vi "Navigation_Main_position_testing april 22.vi"() -> ()   [LabVIEW 2015]
uses:
  <vilib>/myRIO/Instrument Drivers/Onboard IO/PWM/typedefs/PWM Reference.ctl
  <vilib>/myRIO/Common/Instrument Driver Framework/Utilities/typedefs/myRIO Generic Hardware Reference.ctl
  <vilib>/myRIO/Common/Instrument Driver Framework/Utilities/typedefs/Hardware Version Enum.ctl
  <vilib>/myRIO/Common/Instrument Driver Framework/Utilities/typedefs/myRIO v1.0 Reference.ctl
  <vilib>/myRIO/Common/Instrument Driver Framework/Utilities/typedefs/Generic FPGA Reference.ctl
  <vilib>/myRIO/Common/Instrument Driver Framework/myRIO v1.0/PWM/typedefs/PWM Channels Enum.ctl
  <vilib>/myRIO/Instrument Drivers/Onboard IO/PWM/typedefs/PWM Configuration.ctl
  <vilib>/userdefined/High Color/nirio_resource_hc.ctl
  <vilib>/myRIO/Common/Instrument Driver Framework/myRIO v1.0/PWM/vis/myRIO v1.1 Open PWM.vi
  <vilib>/myRIO/Common/Instrument Driver Framework/Utilities/vis/Validate Channels.vi
  <vilib>/myRIO/Common/Instrument Driver Framework/myRIO v1.0/PWM/vis/myRIO v1.0 Reserve PWM.vi
  <vilib>/myRIO/Common/Instrument Driver Framework/myRIO v1.0/PWM/vis/myRIO v1.0 Build MUX Configuration PWM.vi
  <vilib>/myRIO/Common/Instrument Driver Framework/myRIO v1.0/Resource Manager/vis/myRIO v1.0 Reserve Channel List.vi
  <vilib>/myRIO/Common/Instrument Driver Framework/myRIO v1.0/Resource Manager/vis/myRIO v1.0 Create Configuration List.vi
  <vilib>/myRIO/Common/Instrument Driver Framework/myRIO v1.0/Resource Manager/vis/myRIO v1.0 Reserve Channel.vi
  <vilib>/myRIO/Common/Instrument Driver Framework/myRIO v1.0/Resource Manager/vis/myRIO v1.0 Unreserve Channel.vi
  <vilib>/myRIO/Common/Instrument Driver Framework/myRIO v1.0/Resource Manager/vis/myRIO v1.0 Build Mutex Name.vi
  <vilib>/FPGAPlugInAG/myRIO-1900/niLvFpga_Open_myRIO-1900.vi
  <vilib>/rvi/interface/common/dynamic/niFpgaDynamicAddResources.vi
  <vilib>/myRIO/Common/Instrument Driver Framework/Utilities/vis/FPGA Ref Manager.vi
  <vilib>/Utility/error.llb/Error Cluster From Error Code.vi
  <vilib>/myRIO/Common/Instrument Driver Framework/Utilities/vis/Ref Counter.vi
  <vilib>/rvi/errors/niLvFpgaAdjustHostInterfaceError.vi
  <vilib>/Utility/VariantDataType/GetNumericInfo.vi
  <vilib>/myRIO/Common/Instrument Driver Framework/myRIO v1.0/myRIO v1.1 Open.vi
  <vilib>/myRIO/Common/Instrument Driver Framework/Utilities/vis/IO Manager.vi
  <vilib>/myRIO/Common/Instrument Driver Framework/Utilities/vis/Configuration Manager.vi
  <vilib>/myRIO/Common/Instrument Driver Framework/myRIO v1.0/Resource Manager/vis/myRIO v1.0 Configure IO.vi
  <vilib>/myRIO/Common/Instrument Driver Framework/myRIO v1.0/myRIO v1.0 Close.vi
  <vilib>/myRIO/Common/Instrument Driver Framework/myRIO v1.0/PWM/vis/myRIO v1.0 Write PWM.vi
  <vilib>/addons/control/pid/pid.llb/PID (DBL).vi
  <vilib>/rvi/interface/nirviOpenFPGA/nirviOpenFPGA.xnode
  Navi/E/FPGA Bitfiles/NavigationProjec_FPGATarget2_FPGAMainNavigati_PWPHW8gwDxI.lvbitx
  <vilib>/rvi/interface/nirviReadWriteControl/nirviReadWriteControl.xnode
  <vilib>/myRIO/Instrument Drivers/Onboard IO/PWM/vis/myRIO PWM Open.xnode
  <vilib>/myRIO/Instrument Drivers/Onboard IO/PWM/PWM.lvlib
  <vilib>/myRIO/Instrument Drivers/Utilities/Utilities.lvlib
  NiFpgaLv.dll
  <vilib>/rvi/interface/Simulation/niFpgaSimulationCallBeginRW.vi
  <vilib>/addons/control/pid/NI_PID_pid.lvlib
panel:
  in  "camera drop out while loop":bool
  in  "mining control while loop":bool
  in  "Boolean 2":bool=TRUE
  out "stop switch":dbl=1.0
  out "distance to goal":dbl
  out "loc_y":dbl
  out "loc_x":dbl
  out "loc_theta":dbl
  out "start y":dbl
  out "start angle":dbl=1.0
  out "start x":dbl=1.0
  in  "set start position":bool=TRUE
  out "goal reached":bool=TRUE
  out "x/y":dbl
  out "scale":dbl=1.0
  in  "x goal":dbl=10.0
  in  "L Desired Input Velocity (ft/s) 4":dbl(knob) scale=-4.0..4.0
  in  "R Min Linear Velocity (ft/s)  2":dbl=-2.0 format="%#_13g"
  in  "L Min Linear Velocity (ft/s) 9":dbl=-2.0 format="%#_13g"
  in  "R Max Linear Velocity (ft/s) 5":dbl=2.0 format="%#_13g"
  in  "L Max Linear Velocity (ft/s) 5":dbl=2.0 format="%#_13g"
  in  "R Desired Input Velocity (ft/s) 5":dbl(knob) scale=-4.0..4.0
  out "left":dbl
  out "right":dbl
  out "left wheels actual pwm":dbl
  in  "pid reset left":bool
  out "left pwm":dbl(graph)
  out "dt out (s) 3":dbl format="%.3f"
  in  "output range 3":cluster{"output high":dbl, "output low":dbl}={"output high"=0.13333, "output low"=-0.13333} {"output low" format="%.6f"; "output high" format="%.5f"}
  in  "PID gains 3":T1={"proportional gain (Kc)"=0.002, "integral time (Ti, min)"=7e-07, "derivative time (Td, min)"=0.0} {"derivative time (Td, min)" format="%.8f"; "integral time (Ti, min)" format="%.8f"; "proportional gain (Kc)" format="%.8f"}
  out "desired pwm 2":dbl
  out "feedback 2":dbl
  out ".not. x? 3":bool
  out "Elapsed Time (s) 2":dbl caption="Elapsed Time (s)"
  out "x traveled 2":dbl
  out "y traveled 2":dbl
  out "avg 124":dbl
  out "avg 457":dbl
  out "psi dot 2":dbl
  out "distance traveled 2":dbl
  out "y dot 2":dbl
  out "x dot 2":dbl
  out "x position 2":dbl
  out "y position 2":dbl
  out "reset x y 2":dbl
  out "Tick Count(mSec) 2":u32 caption="Tick Count(mSec)"
  in  "start y 2":dbl=3.0
  in  "start x 2":dbl=1.0
  out "right wheels actual pwm":dbl
  in  "pid reset right":bool
  out "right pwm":dbl(graph)
  out "dt out (s) 2":dbl format="%.3f"
  in  "output range 2":cluster{"output high":dbl, "output low":dbl}={"output high"=0.13333, "output low"=-0.13333} {"output low" format="%.6f"; "output high" format="%.5f"}
  in  "PID gains 2":T1={"proportional gain (Kc)"=0.002, "integral time (Ti, min)"=7e-07, "derivative time (Td, min)"=0.0} {"derivative time (Td, min)" format="%.8f"; "integral time (Ti, min)" format="%.8f"; "proportional gain (Kc)" format="%.8f"}
  out "desired pwm":dbl
  out "feedback":dbl
  out ".not. x? 2":bool
  out "Elapsed Time (s)":dbl
  out "LF Rot Velocity (rot/s)":dbl
  out "LM Rot Velocity (rot/s)":dbl
  out "LR Rot Velocity (rot/s)":dbl
  out "RR Rot Velocity (rot/s)":dbl
  out "RM Linear Velocity (rot/s)":dbl
  out "RF Linear Velocity (rot/s)":dbl
  in  "Encoder Reset":bool
  out "SYS.SELECTA":u8 format="%08b"
  out "ENC.B_c.CNTR":i32
  out "ENC.B_b.CNTR":i32
  out "ENC.B_a.CNTR":i32
  out "ENC.A_c.CNTR":i32
  out "ENC.A_b.CNTR":i32
  out "ENC.A_a.CNTR":i32
  in  "R Min Linear Velocity (ft/s)":dbl=-2.0 format="%#_13g"
  in  "R Max Linear Velocity (ft/s)":dbl=2.0 format="%#_13g"
  in  "L Min Linear Velocity (ft/s)":dbl=-2.0 format="%#_13g"
  in  "L Max Linear Velocity (ft/s)":dbl=2.0 format="%#_13g"
  out "Current Rot Velocity (rot/s)":T2(graph)
  # "Motor Control Parameters"
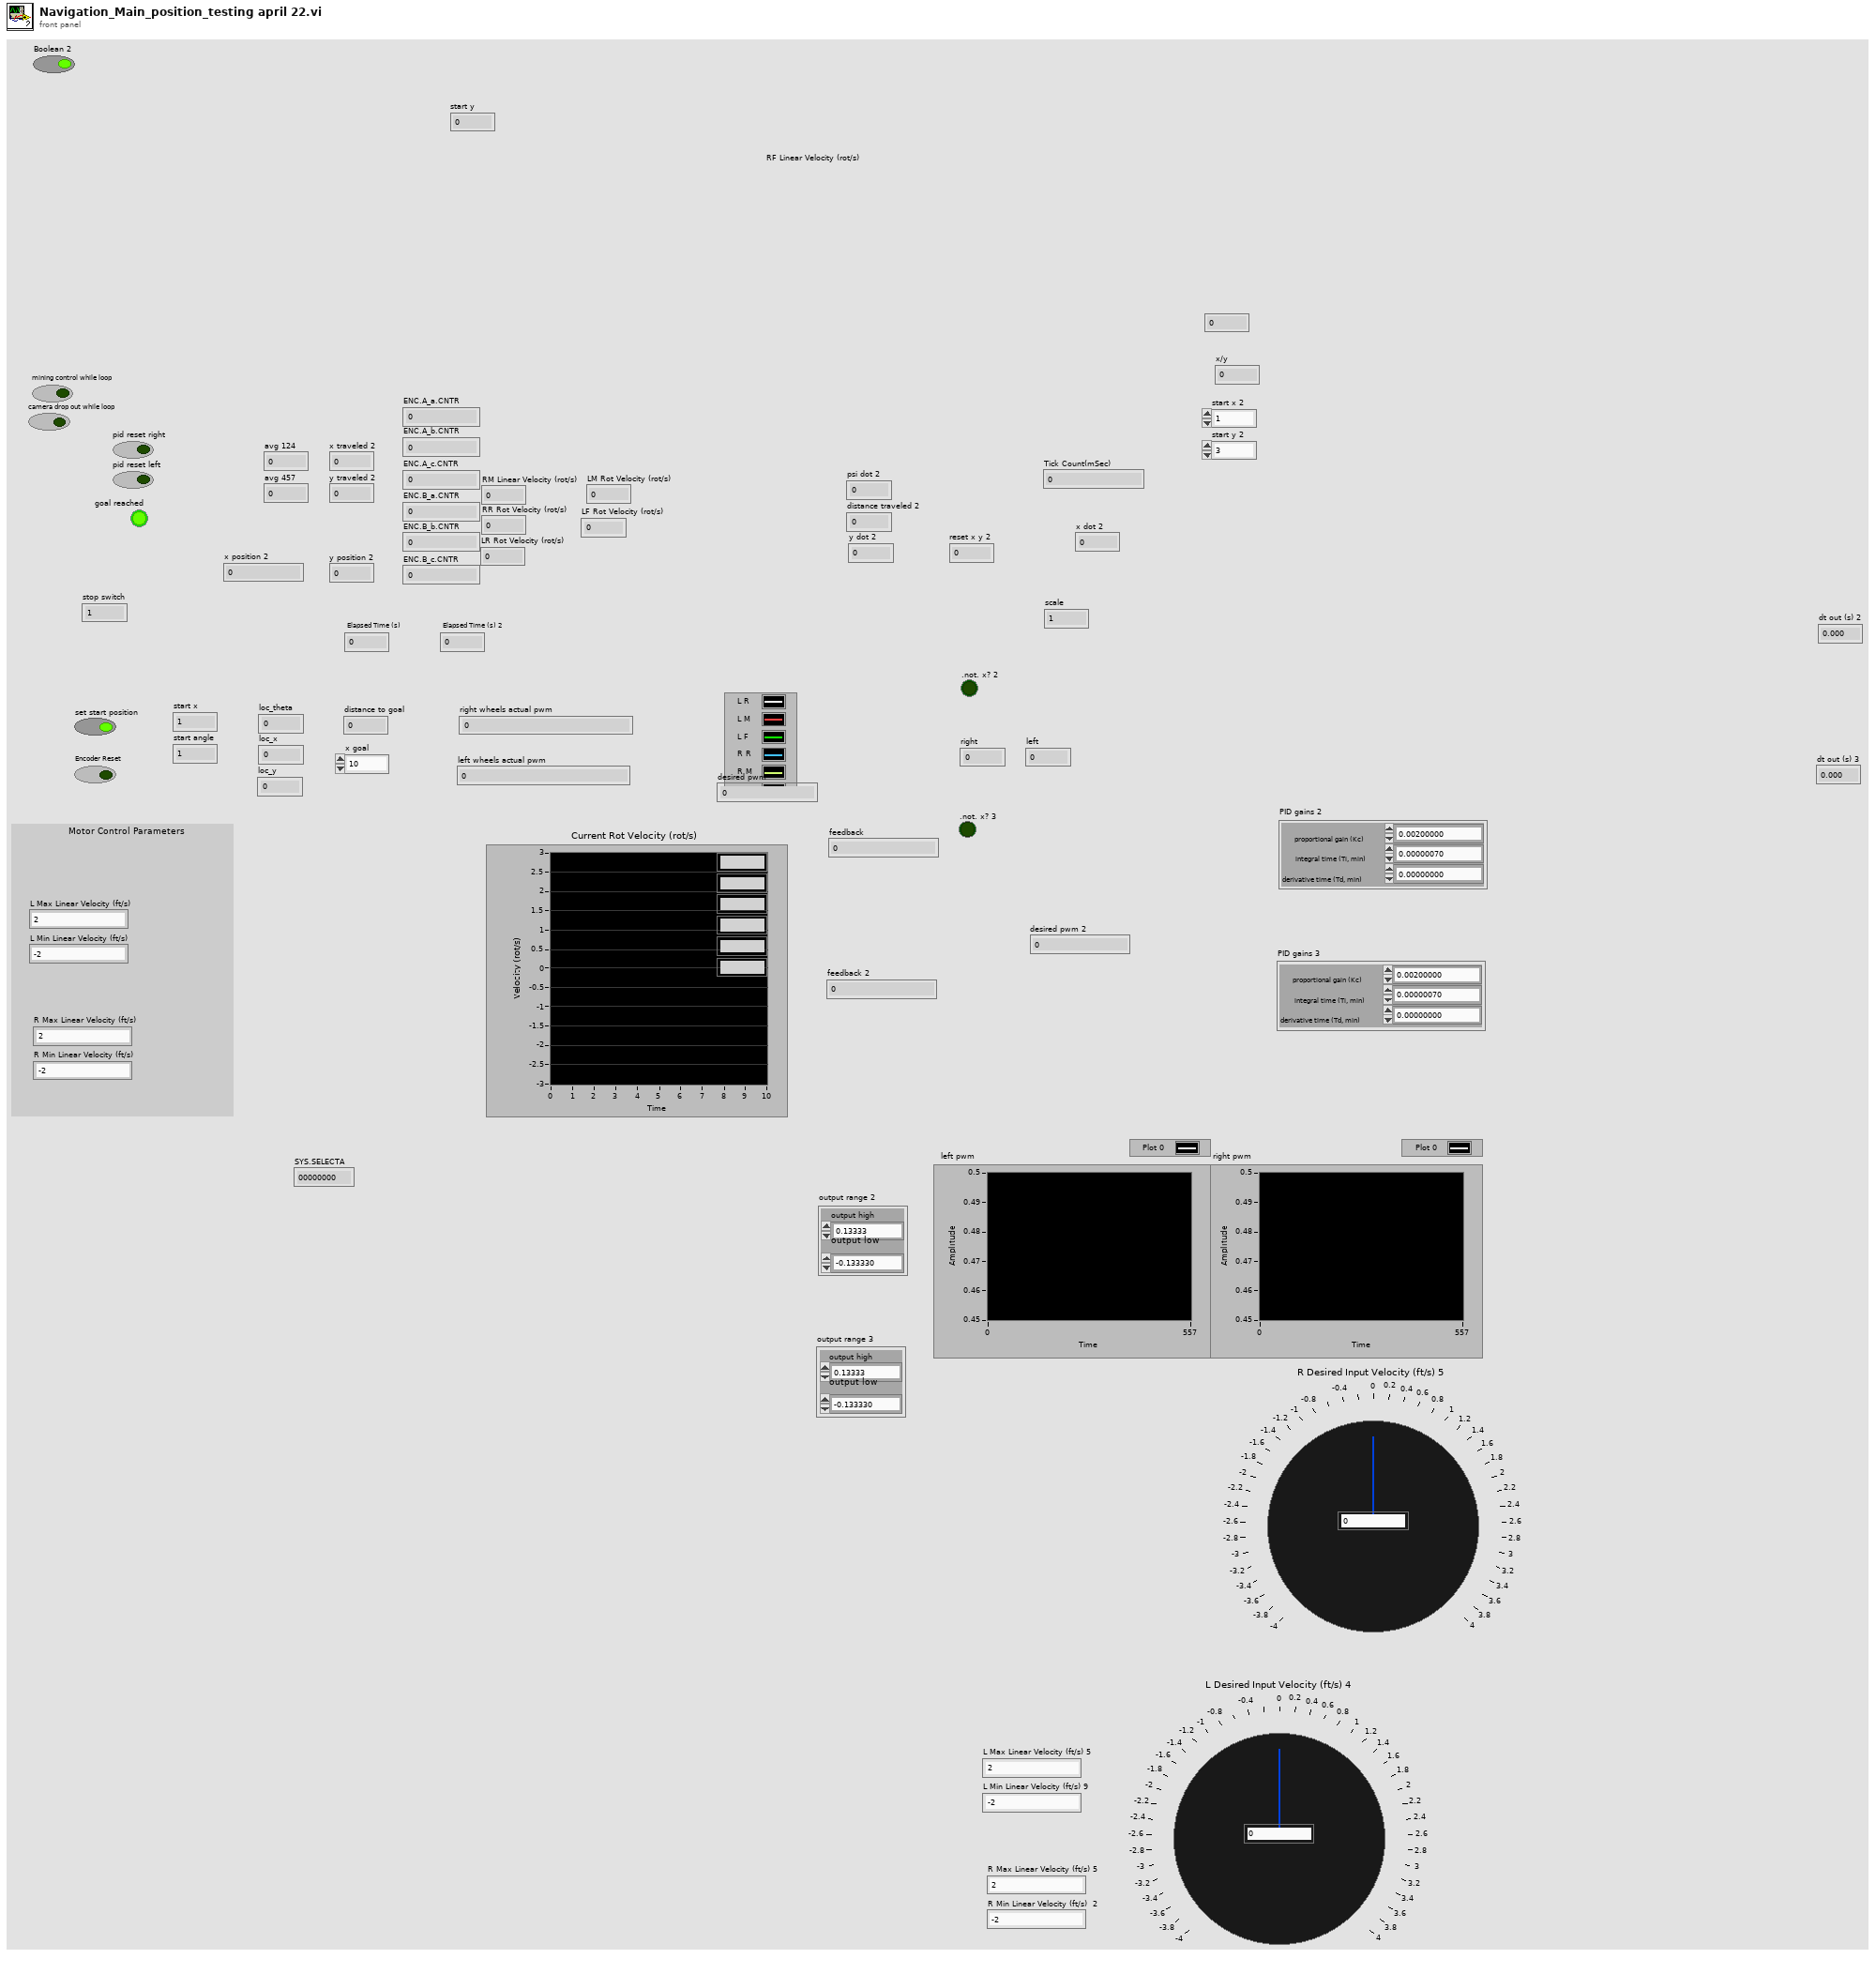
[diagram p1: front panel]
types:
  T1 = cluster{"proportional gain (Kc)":dbl, "integral time (Ti, min)":dbl, "derivative time (Td, min)":dbl}
  T2 = cluster{"Rotational Velocity (RPS)":dbl, "Rotational Velocity (RPS)":dbl, "Rotational Velocity (RPS)":dbl, "Rotational Velocity (RPS)":dbl, "Rotational Velocity (RPS)":dbl, "Rotational Velocity (RPS)":dbl}
  T3 = typedef "nirio_resource_hc.ctl" = tag
  T4 = typedef "Hardware Version Enum.ctl" = enum16{"Unknown", "myRIO-1900", "myRIO-1950", "roboRIO"}
  T5 = typedef "PWM.lvlib/PWM Reference.ctl" = cluster{"myRIO Reference":T6, "PWM Channels Enum":T9, "PWM Configuration":T10}
  T6 = typedef "myRIO Generic Hardware Reference.ctl" = cluster{"myRIO Model":T4, "myRIO Hardware Reference":T7}
  T7 = typedef "myRIO v1.0 Reference.ctl" = cluster{"Generic FPGA Reference":T8, "Allow multiple opens":bool}
  T8 = typedef "Generic FPGA Reference.ctl" = refnum<k20>
  T9 = typedef "PWM Channels Enum.ctl" = enum16{"Not Connected", "C/PWM0", "C/PWM1", "A/PWM0", "A/PWM1", "A/PWM2", "B/PWM0", "B/PWM1", "B/PWM2", "PWM/PWM0", "PWM/PWM1", "PWM/PWM2", "PWM/PWM3", "PWM/PWM4", "PWM/PWM5", "PWM/PWM6", "PWM/PWM7", "PWM/PWM8", "PWM/PWM9"}
  T10 = typedef "PWM.lvlib/PWM Configuration.ctl" = cluster{"Frequency":dbl, "Duty Cycle":dbl}
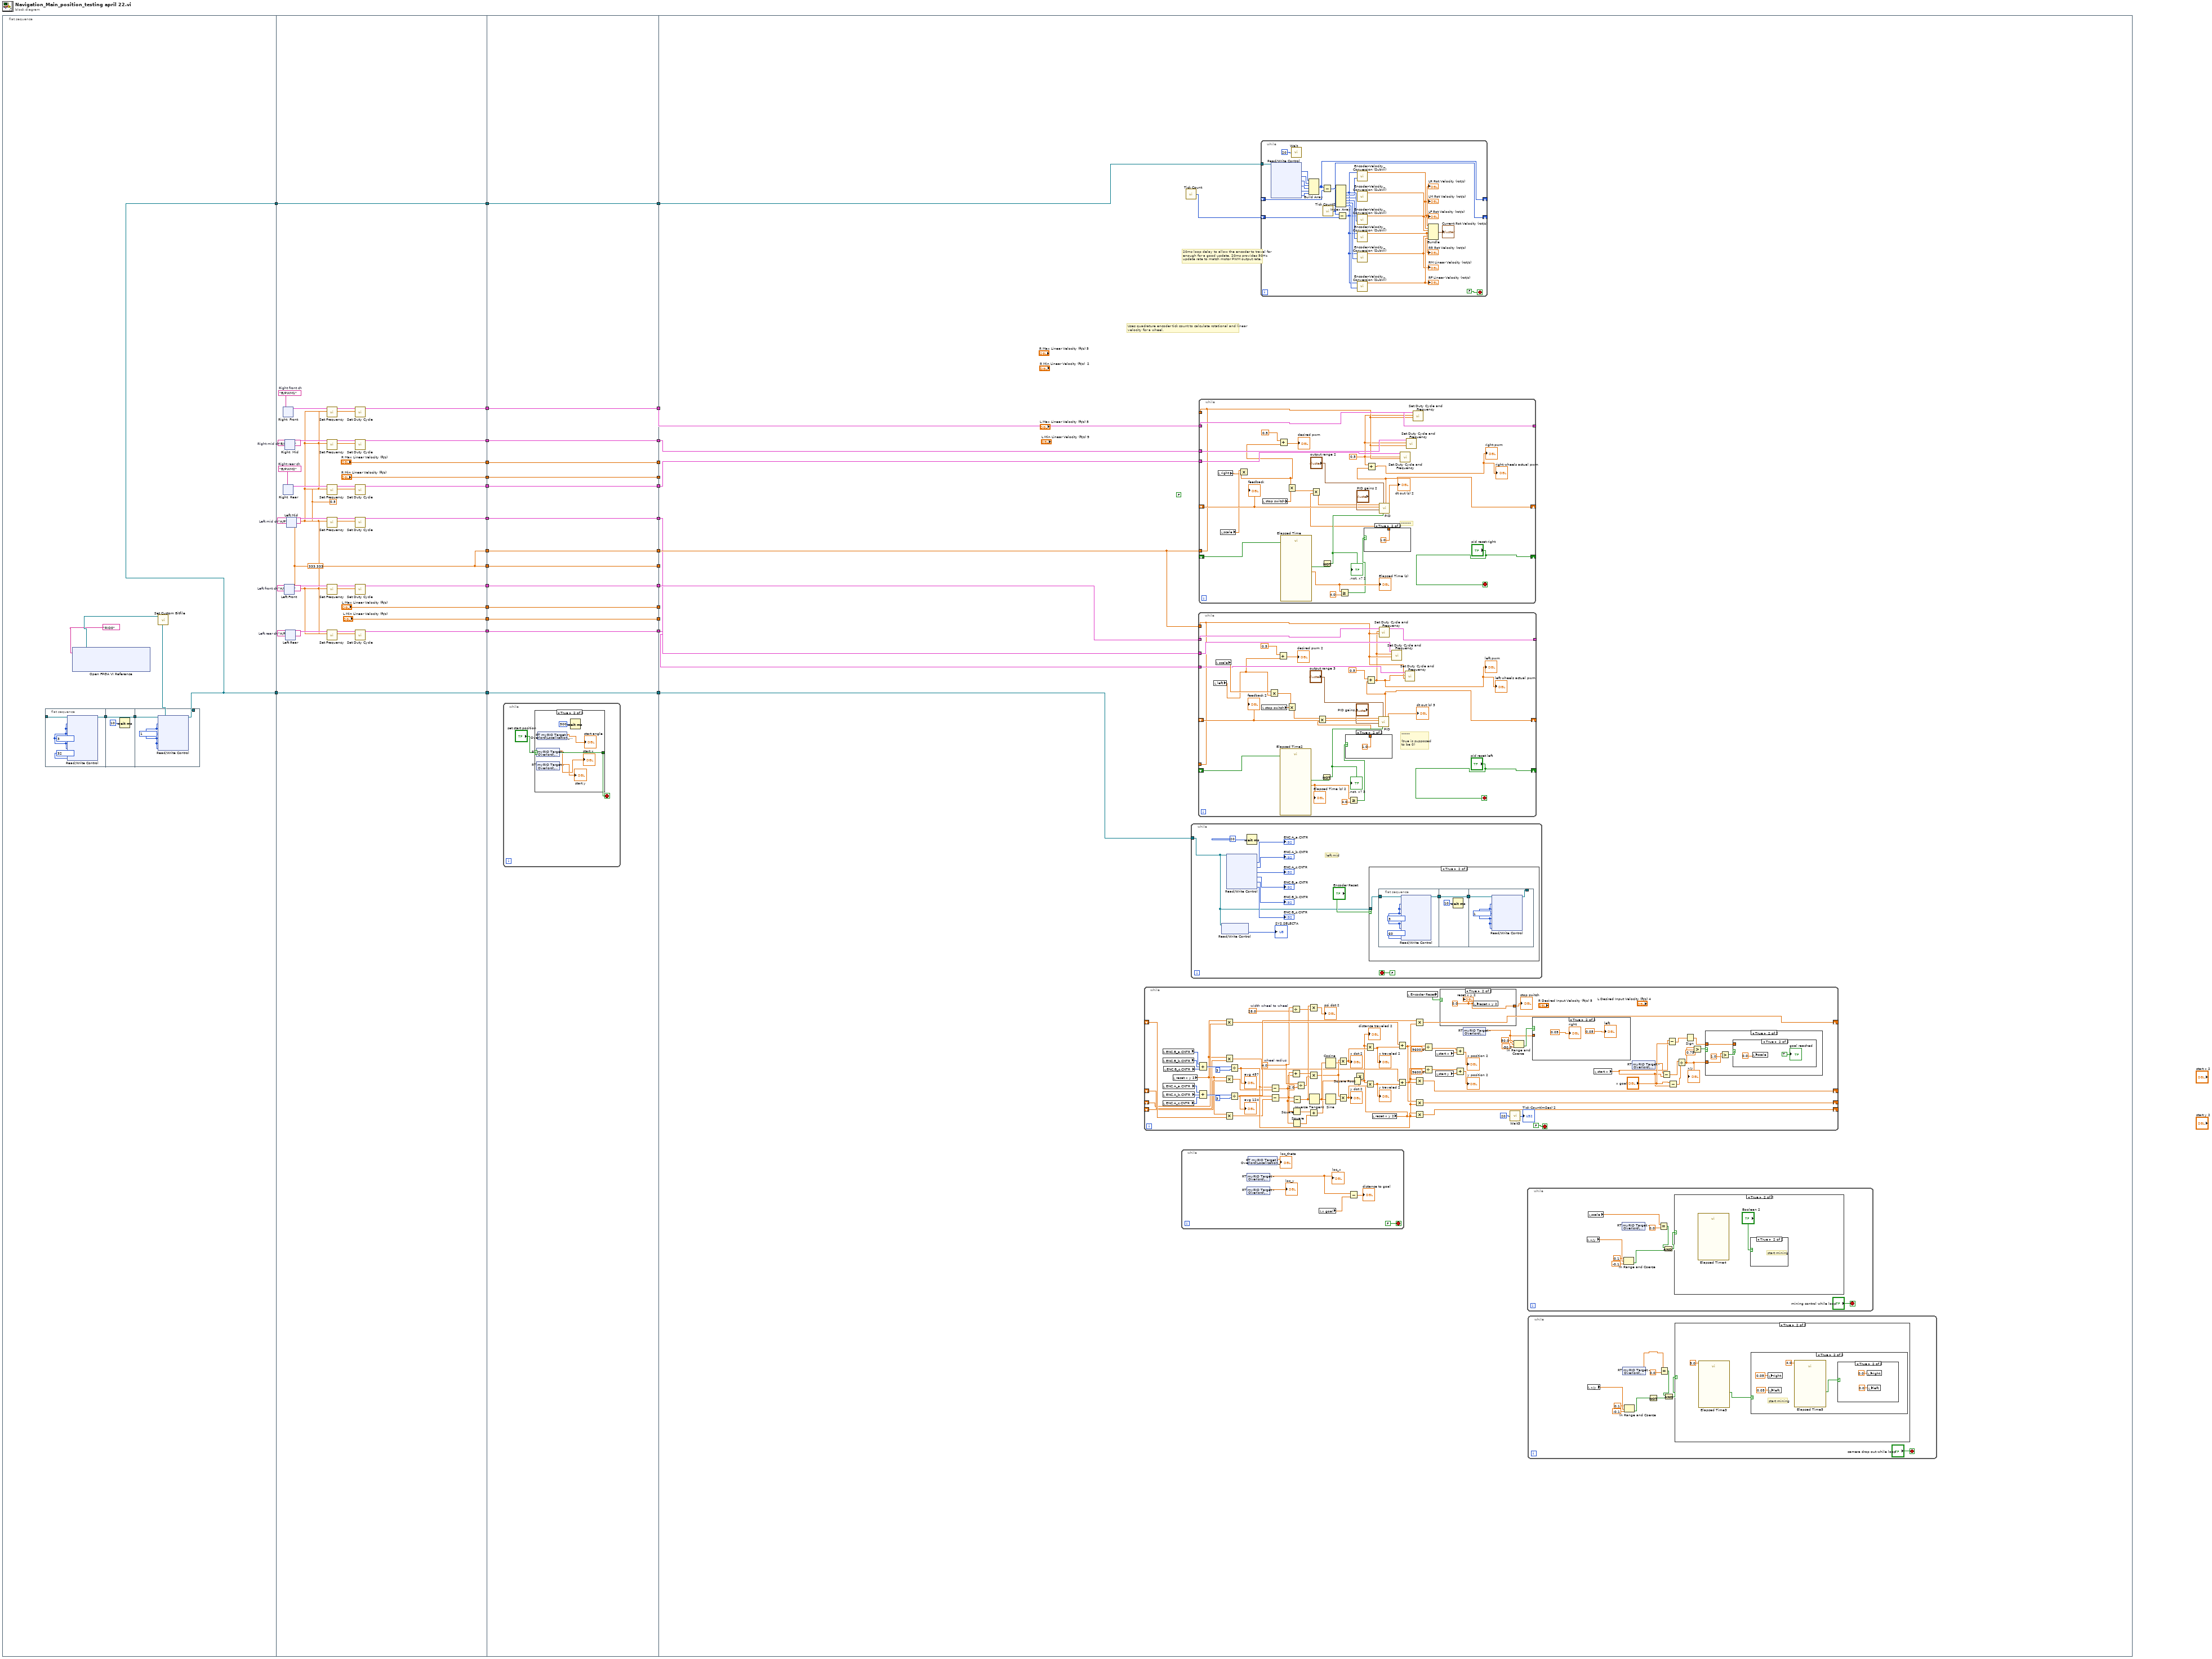
[diagram p0: block diagram]
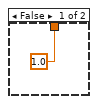
[diagram p8: hidden frame]
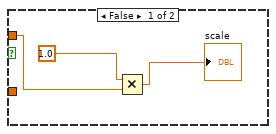
[diagram p9: hidden frame]
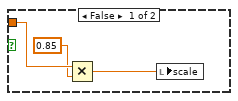
[diagram p10: hidden frame]
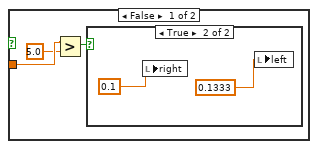
[diagram p11: hidden frame]
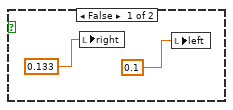
[diagram p12: hidden frame]
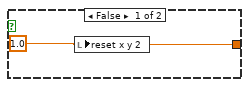
[diagram p13: hidden frame]
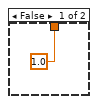
[diagram p14: hidden frame]
diagram:
  n1 = flat-sequence {
    tunnel: [w33] -> w30
    tunnel: [w33] -> w29
    tunnel: [w46] -> w28
    tunnel: [w61] -> w26
    tunnel: [w57] -> w24
    tunnel: [w56] -> w22
    tunnel: [w55] -> w20
    tunnel: [w54] -> w18
    tunnel: [w53] -> w16
    tunnel: ["L Max Linear Velocity (ft/s)"] -> w14
    tunnel: ["L Min Linear Velocity (ft/s)"] -> w12
    tunnel: ["R Max Linear Velocity (ft/s)"] -> w10
    tunnel: ["R Min Linear Velocity (ft/s)"] -> w8
    tunnel: [w48] -> w6
    tunnel: w30 -> [w47]
    tunnel: [w47] -> w4
    tunnel: w29 -> [w48]
    tunnel: [w46] -> w2
    tunnel: w28 -> [w187]
    tunnel: [w187] -> w27
    tunnel: w26 -> [w186]
    tunnel: [w186] -> w25
    tunnel: w24 -> [w185]
    tunnel: [w185] -> w23
    tunnel: w22 -> [w184]
    tunnel: [w184] -> w21
    tunnel: w20 -> [w183]
    tunnel: [w183] -> w19
    tunnel: w18 -> [w182]
    tunnel: [w182] -> w17
    tunnel: w16 -> [w181]
    tunnel: [w181] -> w15
    tunnel: w14 -> [w180]
    tunnel: [w180] -> w13
    tunnel: w12 -> [w179]
    tunnel: [w179] -> w11
    tunnel: w10 -> [w178]
    tunnel: [w178] -> w9
    tunnel: w8 -> [w177]
    tunnel: [w177] -> w7
    tunnel: w6 -> [w176]
    tunnel: [w176] -> w5
    tunnel: w4 -> [w175]
    tunnel: [w175] -> w3
    tunnel: w2 -> [w174]
    tunnel: [w174] -> w1
    tunnel: w27 -> [_]
    tunnel: w25 -> [w195]
    tunnel: w23 -> [w201]
    tunnel: w21 -> [w198]
    tunnel: w19 -> [w197]
    tunnel: w17 -> [w196]
    tunnel: w15 -> [w200]
    tunnel: w13 -> [_]
    tunnel: w11 -> [_]
    tunnel: w9 -> [_]
    tunnel: w7 -> [_]
    tunnel: w5 -> [w203]
    tunnel: w3 -> [w202]
    tunnel: w1 -> [w199]
    frame #0 {
      n2 = flat-sequence {
        tunnel: w34 -> [w39]
        tunnel: [w37] -> w36
        tunnel: w36 -> [w41]
        tunnel: [w41] -> w35
        tunnel: w35 -> [w44]
        tunnel: [w43] -> w33
        frame #0 {
          w38 = u8 32 ("SYS.SELECTA")
          w40 = u8 3 ("ENC.B_c.CNFG")
          n3 = xnode "Read/Write Control"("FPGA VI Reference In"=w39, "ENC.A_a.CNFG"=w40, "ENC.A_b.CNFG"=w40, "ENC.A_c.CNFG"=w40, "ENC.B_a.CNFG"=w40, "ENC.B_b.CNFG"=w40, "ENC.B_c.CNFG"=w40, "SYS.SELECTA"=w38, "SYS.SELECTB"=w38) -> ("FPGA VI Reference Out"=w37:refnum<k20>)  [unwired: 1 in, 1 out]
        }
        frame #1 {
          n4 = Wait (ms)(milliseconds to wait=u32 10) -> ()  [unwired: 1 out]
        }
        frame #2 {
          w45 = u8 1 ("ENC.B_c.CNFG")
          n5 = xnode "Read/Write Control"("FPGA VI Reference In"=w44, "ENC.A_a.CNFG"=w45, "ENC.A_b.CNFG"=w45, "ENC.A_c.CNFG"=w45, "ENC.B_a.CNFG"=w45, "ENC.B_b.CNFG"=w45, "ENC.B_c.CNFG"=w45) -> ("FPGA VI Reference Out"=w43:refnum<k20>)  [unwired: 1 in, 1 out]
        }
      }
      n6 = xnode "Open FPGA VI Reference"("resource name"=tag "RIO0") -> ("FPGA VI Reference Out"=w32:refnum<k20>)  [unwired: 1 in, 1 out]
      n7 = call <vilib>:"Set Custom Bitfile.vi"("Custom FPGA Reference In"=w32) -> ("Custom FPGA Reference Out"=w34:refnum<k20>)  [unwired: 9 in, 1 out]
    }
    frame #1 {
      w58 = 0.5 ("Duty Cycle")
      w46 = 333.333 ("Frequency [Hz]")
      w72 = tag "B/PWM2"  # Right rear ch
      w73 = tag "B/PWM0"  # Right mid ch
      w74 = tag "B/PWM1"  # Right front ch
      w75 = tag "A/PWM2"  # Left rear ch
      w76 = tag "A/PWM1"  # Left mid ch
      w77 = tag "A/PWM0"  # Left front ch
      n8 = xnode "Right  Front"("Channel Name"=w74) -> ("PWM Ref Out"=w68:T5)  [unwired: 2 in, 1 out]
      n9 = xnode "Right  Rear"("Channel Name"=w72) -> ("PWM Ref Out"=w66:T5)  [unwired: 2 in, 1 out]
      n10 = xnode "Left Front"("Channel Name"=w77) -> ("PWM Ref Out"=w71:T5)  [unwired: 2 in, 1 out]
      n11 = xnode "Right  Mid"("Channel Name"=w73) -> ("PWM Ref Out"=w67:T5)  [unwired: 2 in, 1 out]
      n12 = xnode "Left Rear"("Channel Name"=w75) -> ("PWM Ref Out"=w69:T5)  [unwired: 2 in, 1 out]
      n13 = xnode "Left Mid"("Channel Name"=w76) -> ("PWM Ref Out"=w70:T5)  [unwired: 2 in, 1 out]
      n14 = call <vilib>:"Set Frequency.vi"("Frequency [Hz]"=w46, "PWM Ref In"=w68) -> ("PWM Ref Out"=w62:T5)  [unwired: 7 in, 1 out]
      n15 = call <vilib>:"Set Frequency.vi"("Frequency [Hz]"=w46, "PWM Ref In"=w67) -> ("PWM Ref Out"=w63:T5)  [unwired: 7 in, 1 out]
      n16 = call <vilib>:"Set Frequency.vi"("Frequency [Hz]"=w46, "PWM Ref In"=w66) -> ("PWM Ref Out"=w64:T5)  [unwired: 7 in, 1 out]
      n17 = call <vilib>:"Set Frequency.vi"("Frequency [Hz]"=w46, "PWM Ref In"=w70) -> ("PWM Ref Out"=w59:T5)  [unwired: 7 in, 1 out]
      n18 = call <vilib>:"Set Frequency.vi"("Frequency [Hz]"=w46, "PWM Ref In"=w71) -> ("PWM Ref Out"=w65:T5)  [unwired: 7 in, 1 out]
      n19 = call <vilib>:"Set Frequency.vi"("Frequency [Hz]"=w46, "PWM Ref In"=w69) -> ("PWM Ref Out"=w60:T5)  [unwired: 7 in, 1 out]
      n20 = call <vilib>:"Set Duty Cycle.vi"("Duty Cycle"=w58, "PWM Ref In"=w62) -> ("PWM Ref Out"=w57:T5)  [unwired: 7 in, 1 out]
      n21 = call <vilib>:"Set Duty Cycle.vi"("Duty Cycle"=w58, "PWM Ref In"=w63) -> ("PWM Ref Out"=w56:T5)  [unwired: 7 in, 1 out]
      n22 = call <vilib>:"Set Duty Cycle.vi"("Duty Cycle"=w58, "PWM Ref In"=w64) -> ("PWM Ref Out"=w55:T5)  [unwired: 7 in, 1 out]
      n23 = call <vilib>:"Set Duty Cycle.vi"("Duty Cycle"=w58, "PWM Ref In"=w59) -> ("PWM Ref Out"=w54:T5)  [unwired: 7 in, 1 out]
      n24 = call <vilib>:"Set Duty Cycle.vi"("Duty Cycle"=w58, "PWM Ref In"=w65) -> ("PWM Ref Out"=w53:T5)  [unwired: 7 in, 1 out]
      n25 = call <vilib>:"Set Duty Cycle.vi"("Duty Cycle"=w58, "PWM Ref In"=w60) -> ("PWM Ref Out"=w61:T5)  [unwired: 7 in, 1 out]
    }
    frame #2 {
      n26 = while {
        stop <- w188 stop-if-true
        n27 = case shown="True" "set start position" {
          selector: "set start position" -> [_ w194]
          tunnel: [_ w194] -> w188
          frame False {
          }
          frame True {
            n28 = shared-variable "RT myRIO Target - Overlord\\Localization_Variables_r0.lvlib\\loc_x"() -> (→"start x":dbl)  [unwired: 1 in, 1 out]
            n29 = shared-variable "RT myRIO Target - Overlord\\Localization_Variables_r0.lvlib\\loc_y"() -> (→"start y":dbl)  [unwired: 1 in, 1 out]
            n30 = shared-variable "RT myRIO Target - Overlord\\Localization_Variables_r0.lvlib\\loc_theta"() -> (→"start angle":dbl)  [unwired: 1 in, 1 out]
            n31 = Wait (ms)(milliseconds to wait=u32 500) -> ()  [unwired: 1 out]
          }
        }
      }
    }
    frame #3 {
      (unwired) FALSE
      # "Uses quadrature encoder tick count to calculate rotational and linear velocity for a wheel."
      # "20ms loop delay to allow the encoder to travel far enough for a good update. 20ms provides 50Hz update rate to match motor PWM output rate."
      n32 = while {
        shift-right: [w295] -> _
        shift-left: _ -> [w333]
        shift-right: [w292] -> _
        shift-left: _ -> [w332]
        shift-right: [w294] -> _
        shift-left: _ -> [w307]
        shift-right: [w293] -> _
        shift-left: _ -> [w306]
        stop <- FALSE stop-if-true
        w328 = 28.0  # width wheel to wheel
        w329 = 4.0  # wheel radius
        n33 = local read "ENC.B_a.CNTR"() -> (w338:i32)
        n34 = local read "ENC.B_b.CNTR"() -> (w337:i32)
        n35 = local read "ENC.A_a.CNTR"() -> (w341:i32)
        n36 = local read "ENC.A_b.CNTR"() -> (w340:i32)
        n37 = local read "ENC.A_c.CNTR"() -> (w339:i32)
        n38 = local read "ENC.B_c.CNTR"() -> (w336:i32)
        n39 = local read "reset x y 2"() -> (w291:dbl)
        n40 = Compound Arithmetic op=ADD(w338, w337, w336) -> (w344:i32)
        n41 = Compound Arithmetic op=ADD(w341, w340, w339) -> (w345:i32)
        n42 = Multiply(x=w291, y=w306) -> (x*y=w297:dbl)
        n43 = Multiply(x=w291, y=w307) -> (x*y=w298:dbl)
        n44 = Multiply(x=w291, y=w332) -> (x*y=w296:dbl)
        n45 = Multiply(x=w291, y=w333) -> (x*y=w299:dbl)
        n46 = Divide(x=w344, y=3) -> (x/y=w331:dbl)
        "avg 457" <- w331
        n47 = Divide(x=w345, y=3) -> (x/y=w334:dbl)
        "avg 124" <- w334
        n48 = Subtract(x=w331, y=w296) -> (x-y=w321:dbl)
        n49 = Subtract(x=w334, y=w299) -> (x-y=w322:dbl)
        n50 = Divide(x=w329, y=w328) -> (x/y=w324:dbl)
        n51 = Add(x=w322, y=w321) -> (x+y=w326:dbl)
        n52 = Square(x=w322) -> (x^2=w319:dbl)
        n53 = Square(x=w321) -> (x^2=w320:dbl)
        n54 = Subtract(x=w322, y=w321) -> (x-y=w325:dbl)
        n55 = Divide(x=w329, y=2.0) -> (x/y=w327:dbl)
        n56 = Multiply(x=w325, y=w324) -> (x*y=→"psi dot 2":dbl)
        n57 = Multiply(x=w326, y=w327) -> (x*y=w315:dbl)
        n58 = Add(x=w319, y=w320) -> (x+y=w318:dbl)
        n59 = Inverse Tangent(1:w325) -> (0:w323:dbl)
        n60 = Cosine(x=w323) -> (cos(x)=w316:dbl)
        n61 = Sine(x=w323) -> (sin(x)=w317:dbl)
        n62 = Multiply(x=w315, y=w316) -> (x*y=w313:dbl)
        "x dot 2" <- w313
        n63 = Multiply(x=w315, y=w317) -> (x*y=w314:dbl)
        "y dot 2" <- w314
        n64 = Square Root(x=w318) -> (sqrt(x)=w312:dbl)
        n65 = local read "reset x y 2"() -> (w289:dbl)
        n66 = Multiply(x=w312, y=w289) -> (x*y=w290:dbl)
        "distance traveled 2" <- w290
        n67 = Multiply(x=w290, y=w313) -> (x*y=w311:dbl)
        "x traveled 2" <- w311
        n68 = Multiply(x=w290, y=w314) -> (x*y=w310:dbl)
        "y traveled 2" <- w310
        n69 = Add(x=w297, y=w311) -> (x+y=w309:dbl)
        n70 = Add(x=w298, y=w310) -> (x+y=w301:dbl)
        n71 = local read "Encoder Reset"() -> (w288:bool)
        n72 = Multiply(x=w334, y=w289) -> (x*y=w295:dbl)
        n73 = Multiply(x=w289, y=w301) -> (x*y=w294:dbl)
        n74 = Multiply(x=w309, y=w289) -> (x*y=w293:dbl)
        n75 = Multiply(x=w331, y=w289) -> (x*y=w292:dbl)
        n76 = Divide(x=w309, y=9600.0) -> (x/y=w304:dbl)
        n77 = Divide(x=w301, y=9600.0) -> (x/y=w305:dbl)
        n78 = local read "start x"() -> (w302:dbl)
        n79 = local read "start y"() -> (w303:dbl)
        n80 = case shown="True" w288 {
          tunnel: [w368 w369] -> w269
          frame False {
            w368 = 1.0
            n81 = local write "reset x y 2"(w368) -> ()
          }
          frame True {
            w369 = 0.0
            n82 = local write "reset x y 2"(w369) -> ()
            "reset x y 2" <- w369
          }
        }
        "stop switch" <- w269
        n83 = Add(x=w304, y=w302) -> (x+y=→"x position 2":dbl)
        n84 = Add(x=w305, y=w303) -> (x+y=→"y position 2":dbl)
        n85 = shared-variable "RT myRIO Target - Overlord\\Localization_Variables_r0.lvlib\\loc_x"() -> (w271:dbl)  [unwired: 1 in, 1 out]
        n86 = call "Wait3"("Count(mSec)"=u32 20) -> ("Tick Count(mSec)"=→"Tick Count(mSec) 2":u32)
        n87 = In Range and Coerce(upper limit=50.0, x=w271, lower limit=-50.0) -> (In Range?=w282:bool)  [unwired: 1 out]
        n88 = case shown="True" w282 {
          tunnel: w271 -> [w361 _]
          frame False {
            n89 = Greater?(x=w361, y=5.0) -> (0:w359:bool)
            n90 = case shown="True" w359 {
              frame False {
                n91 = local write "right"(0.133) -> ()
                n92 = local write "left"(0.1) -> ()
              }
              frame True {
                n93 = local write "right"(0.1) -> ()
                n94 = local write "left"(0.1333) -> ()
              }
            }
          }
          frame True {
            "right" <- 0.05
            "left" <- 0.05
          }
        }
        n95 = local read "start x"() -> (w273:dbl)
        n96 = shared-variable "RT myRIO Target - Overlord\\Localization_Variables_r0.lvlib\\loc_x"() -> (w270:dbl)  [unwired: 1 in, 1 out]
        n97 = Subtract(x=w270, y=w273) -> (x-y=w278:dbl)
        n98 = Subtract(x=w273, y="x goal") -> (x-y=w275:dbl)
        n99 = Subtract(x="x goal", y=w273) -> (x-y=w277:dbl)
        n100 = Divide(x=w278, y=w277) -> (x/y=w279:dbl)
        "x/y" <- w279
        n101 = Sign(1:w275) -> (0:w274:dbl)
        n102 = Greater?(x=w279, y=0.75) -> (0:w280:bool)
        n103 = case shown="True" w280 {
          tunnel: w279 -> [_ w353]
          tunnel: w274 -> [w348 w350]
          frame False {
            n104 = Multiply(x=1.0, y=w348) -> (x*y=→"scale":dbl)
          }
          frame True {
            n105 = Greater?(x=w353, y=1.0) -> (0:w351:bool)
            n106 = case shown="True" w351 {
              tunnel: w350 -> [w356 _]
              frame False {
                n107 = Multiply(x=w356, y=0.85) -> (x*y=w354:dbl)
                n108 = local write "scale"(w354) -> ()
              }
              frame True {
                n109 = local write "scale"(0.0) -> ()
                "goal reached" <- TRUE
              }
            }
          }
        }
      }
      n110 = while {
        stop <- FALSE stop-if-true
        n111 = shared-variable "RT myRIO Target - Overlord\\Localization_Variables_r0.lvlib\\loc_x"() -> (w236:dbl)  [unwired: 1 in, 1 out]
        "loc_x" <- w236
        n112 = shared-variable "RT myRIO Target - Overlord\\Localization_Variables_r0.lvlib\\loc_y"() -> (→"loc_y":dbl)  [unwired: 1 in, 1 out]
        n113 = shared-variable "RT myRIO Target - Overlord\\Localization_Variables_r0.lvlib\\loc_theta"() -> (→"loc_theta":dbl)  [unwired: 1 in, 1 out]
        n114 = local read "x goal"() -> (w235:dbl)
        n115 = Subtract(x=w236, y=w235) -> (x-y=→"distance to goal":dbl)
      }
      n116 = call "Tick Count"() -> ("Tick Count(uSec)"=w204:u32)
      n117 = while {
        tunnel: w203 -> [w400]
        stop <- FALSE stop-if-true
        # "left mid"
        n118 = xnode "Read/Write Control"("FPGA VI Reference In"=w400) -> ("SYS.SELECTA"=→"SYS.SELECTA":u8)  [unwired: 1 in, 2 out]
        n119 = xnode "Read/Write Control"("FPGA VI Reference In"=w400) -> ("ENC.A_a.CNTR"=→"ENC.A_a.CNTR":u32, "ENC.A_b.CNTR"=→"ENC.A_b.CNTR":u32, "ENC.A_c.CNTR"=→"ENC.A_c.CNTR":u32, "ENC.B_a.CNTR"=→"ENC.B_a.CNTR":u32, "ENC.B_b.CNTR"=→"ENC.B_b.CNTR":u32, "ENC.B_c.CNTR"=→"ENC.B_c.CNTR":u32)  [unwired: 1 in, 2 out]
        n120 = Wait (ms)(milliseconds to wait=u32 20) -> ()  [unwired: 1 out]
        n121 = case shown="True" "Encoder Reset" {
          tunnel: w400 -> [_ w411]
          frame False {
          }
          frame True {
            n122 = flat-sequence {
              tunnel: w411 -> [w416]
              tunnel: [w414] -> w413
              tunnel: w413 -> [w418]
              tunnel: [w418] -> w412
              tunnel: w412 -> [w421]
              tunnel: [w420] -> _
              frame #0 {
                w415 = u8 60 ("SYS.SELECTA")
                w417 = u8 3 ("ENC.B_c.CNFG")
                n123 = xnode "Read/Write Control"("FPGA VI Reference In"=w416, "ENC.A_a.CNFG"=w417, "ENC.A_b.CNFG"=w417, "ENC.A_c.CNFG"=w417, "ENC.B_a.CNFG"=w417, "ENC.B_b.CNFG"=w417, "ENC.B_c.CNFG"=w417, "SYS.SELECTA"=w415, "SYS.SELECTB"=w415) -> ("FPGA VI Reference Out"=w414:refnum<k20>)  [unwired: 1 in, 1 out]
              }
              frame #1 {
                n124 = Wait (ms)(milliseconds to wait=u32 10) -> ()  [unwired: 1 out]
              }
              frame #2 {
                w422 = u8 1 ("ENC.B_c.CNFG")
                n125 = xnode "Read/Write Control"("FPGA VI Reference In"=w421, "ENC.A_a.CNFG"=w422, "ENC.A_b.CNFG"=w422, "ENC.A_c.CNFG"=w422, "ENC.B_a.CNFG"=w422, "ENC.B_b.CNFG"=w422, "ENC.B_c.CNFG"=w422) -> ("FPGA VI Reference Out"=w420:refnum<k20>)  [unwired: 1 in, 1 out]
              }
            }
          }
        }
      }
      n126 = while {
        tunnel: w200 -> [w265]
        tunnel: [w266] -> _
        tunnel: w199 -> [w253]
        shift-right: [w252] -> _
        shift-left: _ -> [w261]
        shift-right: ["pid reset left"] -> _
        shift-left: _ -> [w244]
        tunnel: [w253] -> _
        tunnel: w196 -> [w255]
        tunnel: w195 -> [w254]
        stop <- "pid reset left" stop-if-true
        # "*****\n\n(true is supposed\nto be 0)"
        n127 = local read "left"() -> (w251:dbl)
        n128 = local read "scale"() -> (w256:dbl)
        n129 = local read "stop switch"() -> (w248:dbl)
        n130 = Multiply(x=w256, y=w251) -> (x*y=w250:dbl)
        n131 = Add(x=0.5, y=w251) -> (x+y=→"desired pwm 2":dbl)
        n132 = call "Elapsed Time2"("Reset"=w244) -> ("Elapsed Time (s)"=w243:dbl, "Time has Elapsed"=w247:bool)  [unwired: 11 in, 6 out]
        "Elapsed Time (s) 2" <- w243
        n133 = Multiply(x=w250, y=w248) -> (x*y=w249:dbl)
        n134 = Not(x=w247) -> (.not. x?=w260:bool)
        ".not. x? 3" <- w260
        n135 = Greater Or Equal?(x=w243, y=4.0) -> (x >= y?=w241:bool)
        n136 = case shown="True" w241 {
          tunnel: [1.0 1.0] -> w245
          frame False {
          }
          frame True {
          }
        }
        n137 = Multiply(x=w249, y=w245) -> (x*y=w246:dbl)
        n138 = call-poly <vilib>:"PID.vi"("reinitialize? (F)"=w260, "output range"="output range 3", "PID gains"="PID gains 3", "process variable"=w261, "setpoint"=w246) -> ("dt out (s)"=→"dt out (s) 3":dbl, "output"=w252:dbl)  [unwired: 5 in]
        n139 = Add(x=0.5, y=w252) -> (x+y=w239:dbl)
        "left wheels actual pwm" <- w239
        "left pwm" <- w239
        n140 = call <vilib>:"Set Duty Cycle and Frequency.vi"("Frequency [Hz]"=w253, "Duty Cycle"=w239, "PWM Ref In"=w265) -> ("PWM Ref Out"=w266:T5)  [unwired: 6 in, 1 out]
        n141 = call <vilib>:"Set Duty Cycle and Frequency.vi"("Frequency [Hz]"=w253, "Duty Cycle"=w239, "PWM Ref In"=w255) -> ()  [unwired: 6 in, 2 out]
        n142 = call <vilib>:"Set Duty Cycle and Frequency.vi"("Frequency [Hz]"=w253, "Duty Cycle"=w239, "PWM Ref In"=w254) -> ()  [unwired: 6 in, 2 out]
        "feedback 2" <- w261
      }
      n143 = while {
        tunnel: w201 -> [w396]
        tunnel: [w397] -> _
        tunnel: [w384] -> _
        shift-right: [w383] -> _
        shift-left: _ -> [w392]
        shift-right: ["pid reset right"] -> _
        shift-left: _ -> [w376]
        tunnel: w199 -> [w384]
        tunnel: w198 -> [w386]
        tunnel: w197 -> [w385]
        stop <- "pid reset right" stop-if-true
        w370 = 0.5
        # "******"
        n144 = local read "right"() -> (w382:dbl)
        n145 = local read "scale"() -> (w387:dbl)
        n146 = Multiply(x=w387, y=w382) -> (x*y=w381:dbl)
        n147 = local read "stop switch"() -> (w379:dbl)
        n148 = Add(x=0.5, y=w381) -> (x+y=→"desired pwm":dbl)
        n149 = call "Elapsed Time"("Reset"=w376) -> ("Elapsed Time (s)"=w375:dbl, "Time has Elapsed"=w373:bool)  [unwired: 11 in, 6 out]
        "Elapsed Time (s)" <- w375
        n150 = Multiply(x=w381, y=w379) -> (x*y=w380:dbl)
        n151 = Not(x=w373) -> (.not. x?=w391:bool)
        ".not. x? 2" <- w391
        n152 = Greater Or Equal?(x=w375, y=4.0) -> (x >= y?=w372:bool)
        n153 = case shown="True" w372 {
          tunnel: [1.0 1.0] -> w377
          frame False {
          }
          frame True {
          }
        }
        n154 = Multiply(x=w380, y=w377) -> (x*y=w378:dbl)
        n155 = call-poly <vilib>:"PID.vi"("reinitialize? (F)"=w391, "output range"="output range 2", "PID gains"="PID gains 2", "process variable"=w392, "setpoint"=w378) -> ("dt out (s)"=→"dt out (s) 2":dbl, "output"=w383:dbl)  [unwired: 5 in]
        n156 = Add(x=w370, y=w383) -> (x+y=→"right wheels actual pwm" →"right pwm":dbl)
        n157 = call <vilib>:"Set Duty Cycle and Frequency.vi"("Frequency [Hz]"=w384, "Duty Cycle"=w370, "PWM Ref In"=w385) -> ()  [unwired: 6 in, 2 out]
        n158 = call <vilib>:"Set Duty Cycle and Frequency.vi"("Frequency [Hz]"=w384, "Duty Cycle"=w370, "PWM Ref In"=w386) -> ()  [unwired: 6 in, 2 out]
        n159 = call <vilib>:"Set Duty Cycle and Frequency.vi"("Frequency [Hz]"=w384, "Duty Cycle"=w370, "PWM Ref In"=w396) -> ("PWM Ref Out"=w397:T5)  [unwired: 6 in, 1 out]
        "feedback" <- w392
      }
      n160 = while {
        shift-right: [w441] -> _
        shift-left: _ -> [w440]
        shift-right: [w438] -> _
        shift-left: w204 -> [w437]
        tunnel: w202 -> [w448]
        stop <- FALSE stop-if-true
        n161 = xnode "Read/Write Control"("FPGA VI Reference In"=w448) -> ("ENC.A_a.CNTR"=w447:u32, "ENC.A_b.CNTR"=w446:u32, "ENC.A_c.CNTR"=w445:u32, "ENC.B_a.CNTR"=w444:u32, "ENC.B_b.CNTR"=w443:u32, "ENC.B_c.CNTR"=w442:u32)  [unwired: 1 in, 2 out]
        n162 = call "Wait"("Count(mSec)"=u32 20) -> ()  [unwired: 1 out]
        n163 = Build Array(w447, w446, w445, w444, w443, w442) -> (w441:u32[])
        n164 = Subtract(x=w441, y=w440) -> (x-y=w439:u32[])
        n165 = call "Tick Count2"() -> ("Tick Count(uSec)"=w438:u32)
        n166 = Index Array(array=w439) -> (element #1=w436:u32, element #2=w435:u32, element #3=w434:u32, element #4=w433:u32, element #5=w432:u32, element #6=w431:u32)  [unwired: 6 in]
        n167 = Subtract(x=w438, y=w437) -> (x-y=w430:u32)
        n168 = call "Encoder-Velocity_Conversion (SubVI).vi"("delta  Encoder Count"=w435, "dt (uSec)"=w430) -> ("Rotational Velocity (RPS)"=w425:dbl)  [unwired: 7 in, 2 out]
        "LM Rot Velocity (rot/s)" <- w425
        n169 = call "Encoder-Velocity_Conversion (SubVI).vi"("delta  Encoder Count"=w434, "dt (uSec)"=w430) -> ("Rotational Velocity (RPS)"=w424:dbl)  [unwired: 7 in, 2 out]
        "LF Rot Velocity (rot/s)" <- w424
        n170 = call "Encoder-Velocity_Conversion (SubVI).vi"("delta  Encoder Count"=w436, "dt (uSec)"=w430) -> ("Rotational Velocity (RPS)"=w426:dbl)  [unwired: 7 in, 2 out]
        "LR Rot Velocity (rot/s)" <- w426
        n171 = call "Encoder-Velocity_Conversion (SubVI).vi"("delta  Encoder Count"=w433, "dt (uSec)"=w430) -> ("Rotational Velocity (RPS)"=w423:dbl)  [unwired: 7 in, 2 out]
        "RR Rot Velocity (rot/s)" <- w423
        n172 = call "Encoder-Velocity_Conversion (SubVI).vi"("delta  Encoder Count"=w432, "dt (uSec)"=w430) -> ("Rotational Velocity (RPS)"=w427:dbl)  [unwired: 7 in, 2 out]
        "RM Linear Velocity (rot/s)" <- w427
        n173 = call "Encoder-Velocity_Conversion (SubVI).vi"("delta  Encoder Count"=w431, "dt (uSec)"=w430) -> ("Rotational Velocity (RPS)"=w428:dbl)  [unwired: 7 in, 2 out]
        "RF Linear Velocity (rot/s)" <- w428
        n174 = Bundle("Rotational Velocity (RPS)"=w426, "Rotational Velocity (RPS)"=w425, "Rotational Velocity (RPS)"=w424, "Rotational Velocity (RPS)"=w423, "Rotational Velocity (RPS)"=w427, "Rotational Velocity (RPS)"=w428) -> (→"Current Rot Velocity (rot/s)":T2)  [unwired: 1 in]
      }
      n175 = while {
        stop <- "mining control while loop" stop-if-true
        n176 = local read "x/y"() -> (w209:dbl)
        n177 = local read "scale"() -> (w212:dbl)
        n178 = shared-variable "RT myRIO Target - Overlord\\Localization_Variables_r0.lvlib\\loc_x"() -> ()  [unwired: 1 in, 2 out]
        n179 = In Range and Coerce(upper limit=0.1, x=w209, lower limit=-0.1) -> (In Range?=w206:bool)  [unwired: 1 out]
        n180 = Equal?(x=w212, y=0.0) -> (x = y?=w211:bool)
        n181 = And(x=w211, y=w206) -> (x .and. y?=w210:bool)
        n182 = case shown="True" w210 {
          frame False {
          }
          frame True {
            n183 = call "Elapsed Time4"() -> ()  [unwired: 12 in, 8 out]
            n184 = case shown="True" "Boolean 2" {
              frame False {
              }
              frame True {
                # "start mining"
              }
            }
          }
        }
      }
      n185 = while {
        stop <- "camera drop out while loop" stop-if-true
        n186 = local read "x/y"() -> (w221:dbl)
        n187 = shared-variable "RT myRIO Target - Overlord\\Localization_Variables_r0.lvlib\\loc_x"() -> (w217:dbl)  [unwired: 1 in, 1 out]
        n188 = In Range and Coerce(upper limit=0.1, x=w221, lower limit=-0.1) -> (In Range?=w218:bool)  [unwired: 1 out]
        n189 = Not(x=w218) -> (.not. x?=w216:bool)
        n190 = Equal?(x=w217, y=0.0) -> (x = y?=w223:bool)
        n191 = And(x=w223, y=w216) -> (x .and. y?=w222:bool)
        n192 = case shown="True" w222 {
          frame False {
          }
          frame True {
            n193 = call "Elapsed Time3"("Time Target (s)"=5.0) -> ("Time has Elapsed"=w226:bool)  [unwired: 11 in, 7 out]
            n194 = case shown="True" w226 {
              frame False {
              }
              frame True {
                # "start mining"
                n195 = local write "right"(0.05 ("right")) -> ()
                n196 = local write "left"(0.05 ("left")) -> ()
                n197 = call "Elapsed Time5"("Time Target (s)"=4.0) -> ("Time has Elapsed"=w228:bool)  [unwired: 11 in, 7 out]
                n198 = case shown="True" w228 {
                  frame False {
                  }
                  frame True {
                    n199 = local write "right"(0.0 ("right")) -> ()
                    n200 = local write "left"(0.0 ("left")) -> ()
                  }
                }
              }
            }
          }
        }
      }
    }
  }
